vi "queryForceActuatorInfo.vi"(8 "error in (no error)":errorcluster, 11 "Model in":refnum<class "Model.lvclass">) -> (0 "error out":errorcluster, 3 "Model out":refnum<class "Model.lvclass">)   [LabVIEW 2016, in "Model.lvclass"]
uses:
  Model.lvclass
  Model.lvclass/Model.ctl
  ILCCommunications/ILCCommunications.lvclass/ILCCommunications.ctl
  Common_RT_ILC/ILC/ILC.lvclass/ILC.ctl
  Common_RT_Modbus/ModbusBuffer/ModbusBuffer.lvclass/ModbusBuffer.ctl
  ILCCommunications/reportFAServerID.vi
  ILCCommunications/reportFAServerStatus.vi
  ILCCommunications/reportFAADCScanRate.vi
  ILCCommunications/reportFACalibrationData.vi
  ILCCommunications/reportServerID.vi
  ILCCommunications/reportServerStatus.vi
  ILCCommunications/reportADCScanRate.vi
  ILCCommunications/reportCalibrationData.vi
  Common_RT_ILC/ILC/addReportServerIDFrame.vi
  Common_RT_ILC/ILC/addReportServerStatusFrame.vi
  Common_RT_ILC/ILC/addADCScanRateFrame.vi
  Common_RT_ILC/ILC/getILCData.vi
  Common_RT_ILC/ILC/setILCData.vi
  Common_RT_ILC/ILC/addReportCalibrationDataFrame.vi
  Common_RT_Modbus/ModbusBuffer/writeHeader.vi
  Common_RT_Modbus/ModbusBuffer/writeU8.vi
  Common_RT_Modbus/ModbusBuffer/writeCRC.vi
  Common_RT_Modbus/ModbusBuffer/writeEndOfFrame.vi
  Common_RT_Modbus/ModbusBuffer/writeWaitForRx.vi
  Common_RT_Modbus/ModbusBuffer/writeByteInstruction.vi
  Common_RT_Modbus/ModbusBuffer/calculateCRC.vi
  Common_RT_FAILC/FAILC/FAILC.lvclass
  D:/Code/ts_M1M3Support/Common_RT_ILC/ILC/ILC.lvclass
  ILCCommunications/ILCCommunications.lvclass
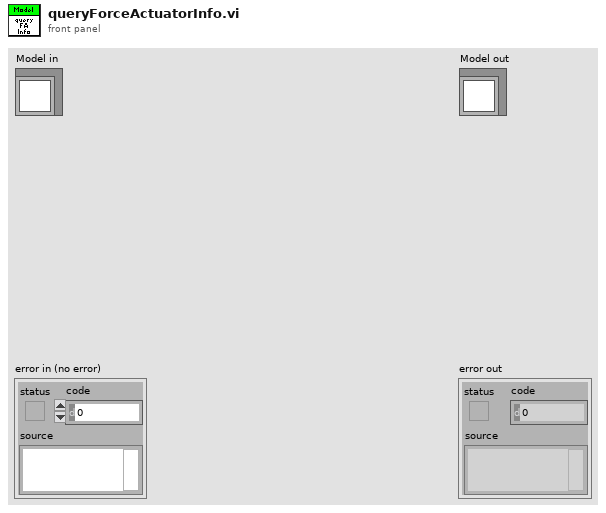
[diagram p1: front panel]
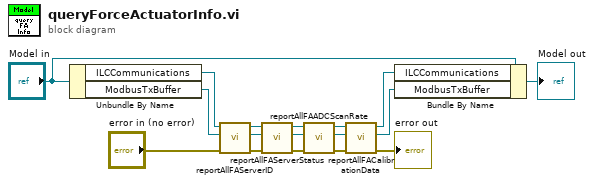
[diagram p0: block diagram]
diagram:
  n1 = Unbundle By Name("Model in") -> ("ILCCommunications"=w15:refnum<class "ILCCommunications.lvclass">, "ModbusTxBuffer"=w10:refnum<class "ModbusBuffer.lvclass">)
  n2 = call "reportAllFAServerID.vi"("error in (no error)"="error in (no error)", "ModbusBuffer in"=w10, "ILCCommunications in"=w15) -> ("error out"=w4:errorcluster, "ModbusBuffer out"=w9:refnum<class "ModbusBuffer.lvclass">, "ILCCommunications out"=w14:refnum<class "ILCCommunications.lvclass">)  [unwired: 6 in]
  n3 = call "reportAllFAServerStatus.vi"("error in (no error)"=w4, "ModbusBuffer in"=w9, "ILCCommunications in"=w14) -> ("error out"=w3:errorcluster, "ModbusBuffer out"=w8:refnum<class "ModbusBuffer.lvclass">, "ILCCommunications out"=w13:refnum<class "ILCCommunications.lvclass">)  [unwired: 6 in]
  n4 = call "reportAllFAADCScanRate.vi"("error in (no error)"=w3, "ModbusBuffer in"=w8, "ILCCommunications in"=w13) -> ("error out"=w2:errorcluster, "ModbusBuffer out"=w7:refnum<class "ModbusBuffer.lvclass">, "ILCCommunications out"=w12:refnum<class "ILCCommunications.lvclass">)  [unwired: 6 in]
  n5 = call "reportAllFACalibrationData.vi"("error in (no error)"=w2, "ModbusBuffer in"=w7, "ILCCommunications in"=w12) -> ("error out"=→"error out":errorcluster, "ModbusBuffer out"=w6:refnum<class "ModbusBuffer.lvclass">, "ILCCommunications out"=w11:refnum<class "ILCCommunications.lvclass">)  [unwired: 6 in]
  n6 = Bundle By Name(cluster="Model in", "ILCCommunications"=w11, "ModbusTxBuffer"=w6) -> (→"Model out":refnum<class "Model.lvclass">)
